vi "Initialize.vi"(8 "error in (no error)":errorcluster, 11 "ATS9350 in":refnum<class "ATS9350.lvclass">) -> (0 "error out":errorcluster, 3 "ATS9350 out":refnum<class "ATS9350.lvclass">)   [LabVIEW 2014, in "ATS9350.lvclass"]
uses:
  ATS9350.lvclass
  ATS-VI/ATS_ctl/Device_Ctrl.ctl
  ATS-VI/ATS_ctl/ATS_Check_Ctrl.ctl
  DAQ Class.lvclass
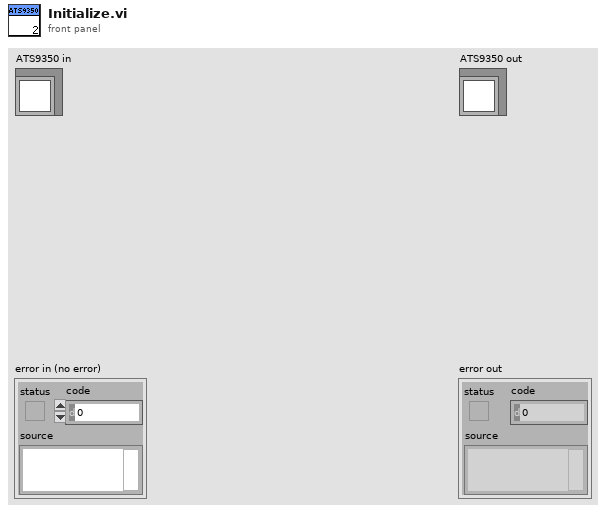
[diagram p1: front panel]
types:
  T1 = typedef "ATS_Check_Ctrl.ctl" = enum16{"None", "NO_ATS9462", "ATS9462_Traditional", "Verify Board", "OnBoard Memory", "Board & Memory", "Master/Slave", "NO Master/Slave"}
  T2 = typedef "Device_Ctrl.ctl" = enum16{"Status", "About", "Arm", "ForceTrig", "Abort", "Initialize", "Init (NoPreset)", "Info", "Close", "Calibrate", "SetManually", "LED_ON", "LED_OFF"}
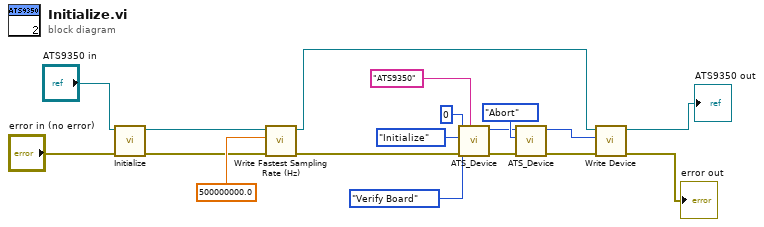
[diagram p0: block diagram]
diagram:
  n1 = call-parent "Initialize.vi"("error in (no error)"="error in (no error)", "DAQ Class in"="ATS9350 in") -> ("error out"=w1:errorcluster, "DAQ Class out"=w2:refnum<class "ATS9350.lvclass">)  [unwired: 8 in]
  n2 = call-dynamic "Write Fastest Sampling Rate (Hz).vi"("error in (no error)"=w1, "Fastest Sampling Rate (Hz)"=500000000.0, "DAQ Class in"=w2) -> ("error out"=w5:errorcluster, "DAQ Class out"=w7:refnum<class "ATS9350.lvclass">)  [unwired: 7 in]
  n3 = call "ATS_Device.vi"("BoardToVerify"="ATS9350", "error in (no error)"=w5, "ATS_Check"=ATS_Check_Ctrl."Verify Board", "DevCtrl"=Device_Ctrl."Initialize", "DeviceIn"=0 ("Device")) -> ("error out"=w11:errorcluster, "DeviceOut"=w14:i32)  [unwired: 5 out]
  n4 = call "ATS_Device.vi"("error in (no error)"=w11, "DevCtrl"=Device_Ctrl."Abort", "DeviceIn"=w14) -> ("error out"=w8:errorcluster, "DeviceOut"=w9:i32)  [unwired: 2 in, 5 out]
  n5 = call-dynamic "Write Device.vi"("error in (no error)"=w8, "Device"=w9, "ATS9350 in"=w7) -> ("error out"=→"error out":errorcluster, "ATS9350 out"=→"ATS9350 out":refnum<class "ATS9350.lvclass">)  [unwired: 7 in]
